vi "generador.vi"() -> ()   [LabVIEW 2017]
uses:
  <vilib>/measure/NI_MABase.lvlib
panel:
  out "Fs":dbl format="%#_13g"
  in  "Boolean":bool=TRUE
  out "Numeric":dbl format="%#_13g"
  out "Nyquist eqn":string
  out "Cycle of signals":i32
  in  "signal type":T1(ring)
  in  "square wave duty cycle (%)":dbl
  in  "Amplitude noise":dbl(knob) min=0.0 max=5.0 step=0.1 scale=0.01..5.0
  in  "Phase":dbl(slide) scale=0.0..10.0
  in  "Amplitude":dbl(knob)=10.0 min=0.1 max=10.0 step=0.1 scale=0.01..10.0
  in  "frequency":dbl(knob)=10000.0 min=100.0 max=10000.0 step=10.0 scale=100.0..10000.0
  in  "offset":dbl(slide) scale=0.0..10.0
  in  "stop":bool
  in  "sampling info":cluster{"Fs":dbl, "#s":dbl}={"Fs"=1000.0, "#s"=1000.0} {"Fs" format="%.2p"}
  out "Waveform Graph":waveform(dbl)(graph)
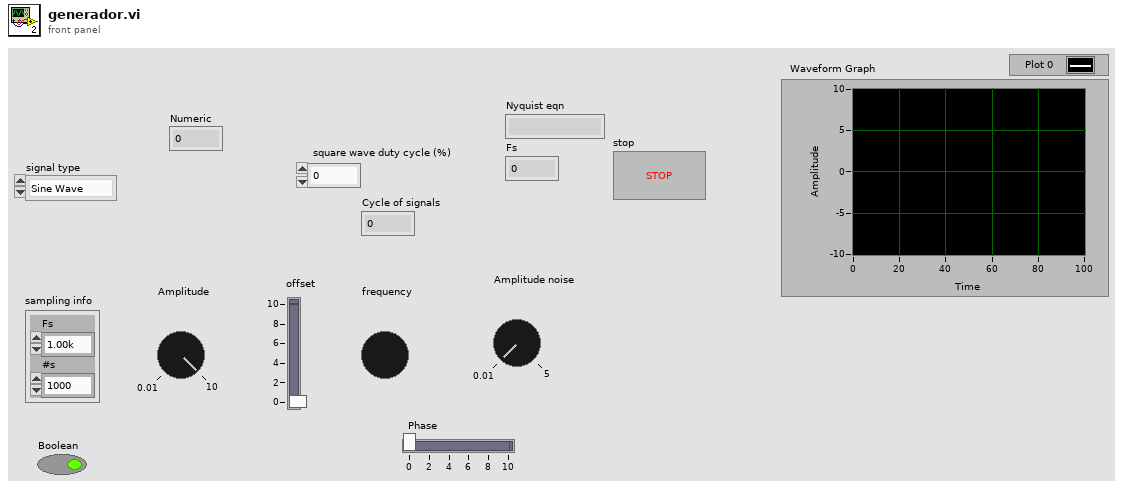
[diagram p1: front panel]
types:
  T1 = enum16{"Sine Wave", "Triangle Wave", "Square Wave", "Sawtooth Wave"}
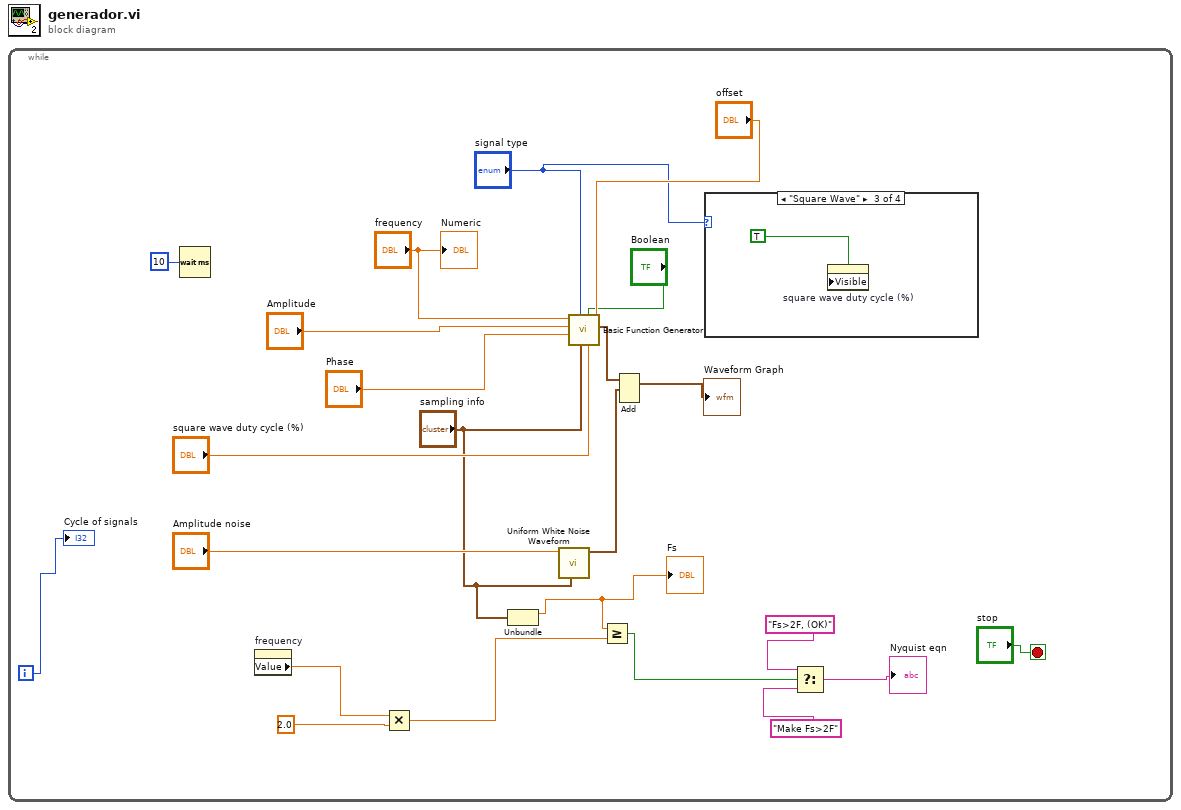
[diagram p0: block diagram]
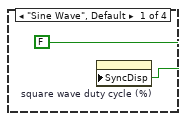
[diagram p2: hidden frame]
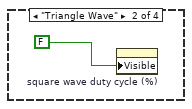
[diagram p3: hidden frame]
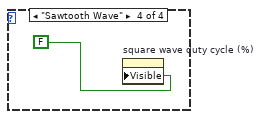
[diagram p4: hidden frame]
diagram:
  n1 = while {
    i -> [w11]
    stop <- "stop" stop-if-true
    n2 = Wait (ms)(milliseconds to wait=u32 10) -> ()  [unwired: 1 out]
    n3 = property on="frequency" class="Knob (strict)"() -> ("Value"=w4:dbl)  [unwired: 2 in, 2 out]
    n4 = Multiply(x=w4, y=2.0) -> (x*y=w6:dbl)
    n5 = Unbundle("sampling info") -> ("Fs"=w1:dbl)  [unwired: 1 out]
    "Fs" <- w1
    n6 = call <vilib>:"Uniform White Noise Waveform.vi"("sampling info"="sampling info", "amplitude"="Amplitude noise") -> ("signal out"=w19:waveform(dbl))  [unwired: 8 in, 1 out]
    n7 = call <vilib>:"Basic Function Generator.vi"("offset"="offset", "square wave duty cycle (%)"="square wave duty cycle (%)", "reset signal"="Boolean", "sampling info"="sampling info", "signal type"="signal type", "phase"="Phase", "amplitude"="Amplitude", "frequency"="frequency") -> ("signal out"=w18:waveform(dbl))  [unwired: 1 in, 2 out]
    n8 = Greater Or Equal?(x=w1, y=w6) -> (x >= y?=w7:bool)
    n9 = Add(1:w19, 2:w18) -> (0:→"Waveform Graph":waveform(dbl))  [unwired: 1 in, 1 out]
    n10 = case shown="\"Square Wave\"" "signal type" {
      frame "Sine Wave", Default {
        n11 = property on="square wave duty cycle (%)" class="DigNum (strict)"("SyncDisp"=FALSE) -> ()  [unwired: 2 in, 2 out]
      }
      frame "Triangle Wave" {
        n12 = property on="square wave duty cycle (%)" class="DigNum (strict)"("Visible"=FALSE) -> ()  [unwired: 2 in, 2 out]
      }
      frame "Square Wave" {
        n13 = property on="square wave duty cycle (%)" class="DigNum (strict)"("Visible"=TRUE) -> ()  [unwired: 2 in, 2 out]
      }
      frame "Sawtooth Wave" {
        n14 = property on="square wave duty cycle (%)" class="DigNum (strict)"("Visible"=FALSE) -> ()  [unwired: 2 in, 2 out]
      }
    }
    n15 = Select(t="Fs>2F, (OK)", s=w7, f="Make Fs>2F") -> (s? t:f=→"Nyquist eqn":string)
    "Cycle of signals" <- w11
    "Numeric" <- "frequency"
  }
